vi "Manual Label Print.vi"(8 "error in (no error)":errorcluster) -> (0 "error out":errorcluster)   [LabVIEW 2017]
panel:
  out "FINAL BARCODE":string
  in  "NO OF PRINT":u16=1 min=1 max=100 step=1
  in  "stop":bool
  in  "Print":bool
  out "VARIENT":string
  out "USER":string
  # "MANUAL LABEL PRINT"
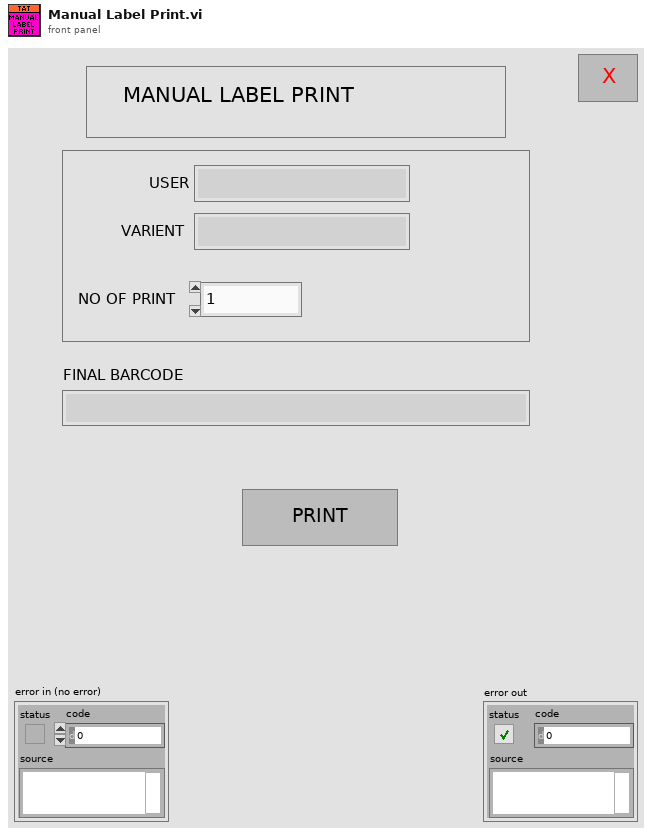
[diagram p1: front panel]
types:
  T1 = typedef "Recipe.ctl" = cluster{"Ass. Sensor Select":cluster{"Ass. Sensor Select":bool, "Camera-1 \nProg No.":u16, "Camera-2 \nProg No.":u16, "Gun \nProg No.":u16}, "Torque Sensor Select":cluster{"Torque Sensor-1":bool, "Torque Sensor-2":bool, "Torque Sensor-3":bool, "Torque Sensor-4":bool, "Torque Sensor-5":bool, "Torque Sensor-6":bool, "Torque Sensor-7":bool, "Torque Sensor-8":bool, "Torque Sensor-9":bool, "Torque Sensor-10":bool, "Torque Sensor-11":bool, "Torque Sensor-12":bool}, "Bin Seq. Select":cluster{"First Bin":u16, "Second Bin":u16, "Third Bin":u16, "Fourth Bin":u16, "Fifth Bin":u16, "Sixth Bin":u16, "Seventh Bin":u16, "Eighth Bin":u16, "Camera-1 Trig":u16, "Camera-2 Trig":u16}, "T-Bin Seq. Select":cluster{"First":u16, "Second":u16, "Third":u16, "Fourth":u16, "Fifth":u16, "Sixth":u16}, "Reference Barcode":cluster{"Spring Barcode":string, "Body Barcode":string, "14 Char of Barcode":string, "Final Barcode Length":string}, "Label Data":cluster{"Cust. Part No.":string, "TML Part No.":string, "Vendor Code":string, "Revision Level":string, "Part Description":string, "Vendor Name":string}}
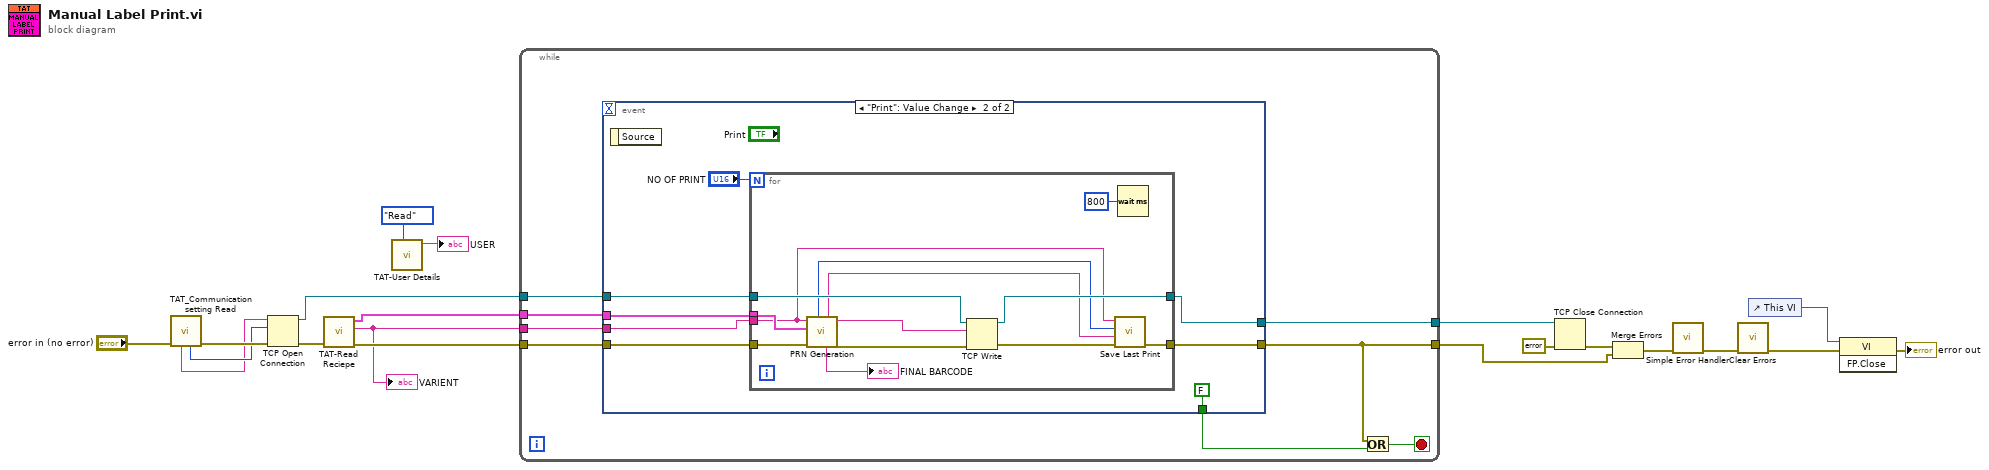
[diagram p0: block diagram]
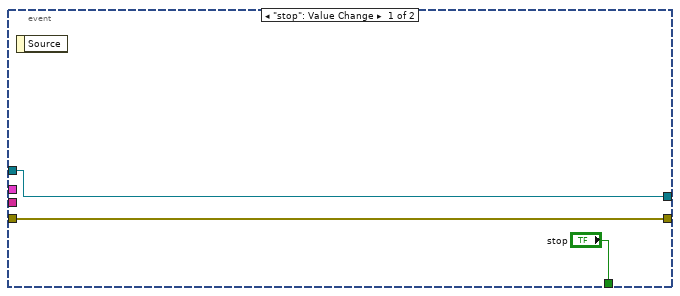
[diagram p2: hidden frame]
diagram:
  n1 = call "TAT_Communication setting Read.vi"("error in (no error)"="error in (no error)") -> ("error out"=w3:errorcluster, "Printer Port"=w2:u32, "Printer IP"=w1:string)  [unwired: 3 in, 5 out]
  n2 = TCP Open Connection(address=w1, remote port or service name=w2, error in (no error)=w3) -> (connection ID=w16:refnum<k5>, error out=w4:errorcluster)  [unwired: 2 in]
  n3 = call "TAT-Read Reciepe.vi"("error in (no error)"=w4) -> ("error out"=w18:errorcluster, "Part Name"=w15:string, "Data To Load"=w17:T1)  [unwired: 8 in]
  "VARIENT" <- w15
  n4 = call "TAT-User Details.vi"("Enum"=enum16{"Read", "Write"}."Read") -> ("User Name Out"=→"USER":string)  [unwired: 9 in, 1 out]
  n5 = while {
    tunnel: w18 -> [w25]
    tunnel: w17 -> [w27]
    tunnel: w16 -> [w26]
    tunnel: w15 -> [w24]
    tunnel: [w22] -> w11
    tunnel: [w21] -> w5
    stop <- w23 stop-if-true
    n6 = event shown="[1] \"Print\": Value Change" {
      selector: _ -> [_ _]
      dyn-events: _ -> [_ _]
      timeout: _ -> [_ _]
      tunnel: ["stop" FALSE ("stop")] -> w28
      tunnel: w27 -> [_ w37]
      tunnel: w26 -> [w29 w36]
      tunnel: w25 -> [w30 w38]
      tunnel: w24 -> [_ w33]
      tunnel: [w30 w34] -> w22
      tunnel: [w29 w35] -> w21
      event "stop": Value Change {
        n7 = event-data() -> ()  [unwired: 1 in, 1 out]
      }
      event "Print": Value Change {
        n8 = event-data() -> ()  [unwired: 1 in, 1 out]
        n9 = for {
          N: "NO OF PRINT" -> [_]
          tunnel: w37 -> [w51]
          tunnel: w33 -> [w43]
          tunnel: w36 -> [w48]
          tunnel: [w46] -> w35
          tunnel: w38 -> [w52]
          tunnel: [w44] -> w34
          n10 = call "PRN Generation.vi"("error in (no error)"=w52, "Ref Data"=w51, "File Name"=w43) -> ("error out"=w49:errorcluster, "PRN to Print"=w47:string, "Barcode"=→"FINAL BARCODE":string, "Printing Date"=w41:string, "SN"=w42:u32)  [unwired: 3 in, 1 out]
          n11 = TCP Write(connection ID=w48, data in=w47, error in (no error)=w49) -> (connection ID out=w46:refnum<k5>, error out=w45:errorcluster)  [unwired: 1 in, 1 out]
          n12 = call "Save Last Print.vi"("error in (no error)"=w45, "Printing Date"=w41, "SN"=w42, "Part Name"=w43) -> ("error out"=w44:errorcluster)  [unwired: 7 in]
          n13 = Wait (ms)(milliseconds to wait=u32 800) -> ()  [unwired: 1 out]
        }
      }
    }
    n14 = Or(x=w22, y=w28) -> (x .or. y?=w23:bool)
  }
  n15 = TCP Close Connection(connection ID=w5, error in (no error)=errorcluster {"status"=FALSE, "code"=0, "source"=""}) -> (error out=w12:errorcluster)  [unwired: 1 in, 1 out]
  n16 = Merge Errors(w12, w11) -> (w10:errorcluster)
  n17 = call <vilib>:"Simple Error Handler.vi"("error in (no error)"=w10) -> ("error out"=w9:errorcluster)  [unwired: 4 in, 4 out]
  n18 = call <vilib>:"Clear Errors.vi"("error in (no error)"=w9) -> ("error out"=w8:errorcluster)  [unwired: 5 in, 1 out]
  n19 = control-ref of="This VI"() -> (w7:refnum<vi>)
  n20 = invoke class="VI" method="FP.Close"(reference=w7, error in=w8) -> (error out=→"error out":errorcluster)  [unwired: 1 in, 2 out]
